vi "Measure.vi"(8 "error in (no error)":errorcluster, 9 "measurement configuration":variant, 10 "measure call context in":refnum<class "Measure Call Context.lvclass">, 11 "measurement plugin in":refnum<class "FPT NoiseFigure.lvclass">) -> (0 "error out":errorcluster, 1 "measurement results":variant, 2 "measure call context out":refnum<class "Measure Call Context.lvclass">, 3 "measurement plugin out":refnum<class "FPT NoiseFigure.lvclass">)   [LabVIEW 2023, in "FPT NoiseFigure.lvclass"]
uses:
  FPT NoiseFigure.lvclass
  <vilib>/Plug-In SDKs/Measurements/Measure Call Context/Measure Call Context.lvclass
  Measurement Configuration.ctl
  FPT NoiseFigure.lvclass/FPT NoiseFigure.ctl
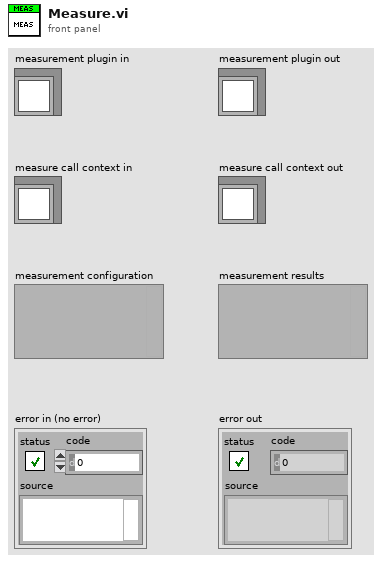
[diagram p1: front panel]
types:
  T1 = typedef "FPT NoiseFigure.lvclass/Measurement Configuration.ctl" = cluster{"Automation Test":bool, "Power sequencing file path":string, "RFmx name":string, "RFmx port":string, "DUT Max Gain (dB)":dbl, "DUT Max Noise Figure (dB)":dbl, "Reference Level Mode":enum32{"Manual", "Recommend"}, "Reference Level (dBm)":dbl, "Preamp Enabled":i32, "RFmx attenuation mode":enum32{"<None>", "Constant Attenuation", "s2p File"}, "RFmx external attenuation (dB)":dbl, "RFmx s-parameters orientation":enum32{"Port1 Towards DUT", "Port2 Towards DUT"}, "RFmx s2p file path":string, "Switch Name":string, "Switch Connection":string, "ENS SMU Name":string, "ENS SMU Channel":string, "Action":u32, "Measurement Bandwidth (Hz)":dbl, "Measurement Interval (s)":dbl, "NF Cal Setup ID":string, "DUT Type":i32, "Frequency List Mode":enum32{"Step", "Points", "Frequency List"}, "Step - Start Frequency ":dbl, "Step - Stop Frequency":dbl, "Step - Step Size":dbl, "Points - Start Frequency":dbl, "Points - Stop Frequency":dbl, "Points - Number of Points":i32, "FreqList - Frequency List":dbl[], "Averaging Enabled":bool, "Averaging Count":i32, "Noise Source Type":i32, "Noise Source RFSG Port":string, "Noise Source Cold Temperature (K)":dbl, "Noise Source Off Temperature (K)":dbl, "ENR Freq (Hz)":dbl[], "ENR (dB)":dbl[], "DUT Input_Compensation Enabled":bool, "DUT Input_Temperation (K)":dbl, "DUT Input_Loss Freq (Hz)":dbl[], "DUT Input_Loss (dB)":dbl[], "DUT Output_Compensation Enabled":bool, "DUT Output_Temperation (K)":dbl, "DUT Output_Loss Freq (Hz)":dbl[], "DUT Output_Loss (dB)":dbl[], "Calibration_Compensation Enabled":bool, "Calibration_Temperation (K)":dbl, "Calibration_Loss Freq (Hz)":dbl[], "Calibration_Loss (dB)":dbl[], "Noise Source_Compensation Enabled":bool, "Noise Source_Temperation (K)":dbl, "Noise Source_Loss Freq (Hz)":dbl[], "Noise Source_Loss (dB)":dbl[], "DUT Input Loss S2P File Path":string, "DUT Input Loss S-Parameter Orientation":i32, "DUT Output Loss S2P File Path":string, "DUT Output Loss S-Parameter Orientation":i32, "Calibration Loss S2P File Path":string, "Calibration Loss S-Parameter Orientation":i32, "Noise Source Loss S2P File Path":string, "Noise Source Loss S-Parameter Orientation":i32, "Power sequencing file validity check":bool}
  T2 = typedef "FPT NoiseFigure.lvclass/Measurement Results.ctl" = cluster{"Status":string, "DUT NF vs Freq":dbl[][], "Analyzer NF vs Freq":dbl[][], "DUT NF (mean)":dbl, "Analyzer NF (mean)":dbl}
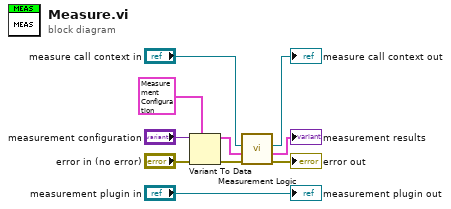
[diagram p0: block diagram]
diagram:
  n1 = Variant To Data(error in="error in (no error)", type=T1 {"Automation Test"=FALSE, "Power sequencing file path"="Lorem ipsum dolor sit", "RFmx name"="5842_0", "RFmx port"="Lorem ipsum dolor sit", "DUT Max Gain (dB)"=3.0, "DUT Max Noise Figure (dB)"=1.2, "Reference Level Mode"=enum."Manual", "Reference Level (dBm)"=1.2, "Preamp Enabled"=0, "RFmx attenuation mode"=enum."Constant Attenuation", "RFmx external attenuation (dB)"=1.0, "RFmx s-parameters orientation"=enum."Port2 Towards DUT", "RFmx s2p file path"="", "Switch Name"="2599_S8", "Switch Connection"="no0->com0", "ENS SMU Name"="", "ENS SMU Channel"="", "Action"=0, "Measurement Bandwidth (Hz)"=4000000.0, "Measurement Interval (s)"=0.1, "NF Cal Setup ID"="SNS_PS_6dB_ENR15_26.5GHz_VI", "DUT Type"=0, "Frequency List Mode"=enum."Step", "Step - Start Frequency "=1000000000.0, "Step - Stop Frequency"=2000000000.0, "Step - Step Size"=100000000.0, "Points - Start Frequency"=1000000000.0, "Points - Stop Frequency"=2000000000.0, "Points - Number of Points"=11, "FreqList - Frequency List"=[4000000000.0, 5000000000.0, 6000000000.0, 7000000000.0, 8000000000.0, 9000000000.0, 10000000000.0, 11000000000.0, 12000000000.0, 13000000000.0, 14000000000.0, 15000000000.0, 16000000000.0, 17000000000.0, 18000000000.0, 19000000000.0, 20000000000.0], "Averaging Enabled"=FALSE, "Averaging Count"=10, "Noise Source Type"=1, "Noise Source RFSG Port"="port1", "Noise Source Cold Temperature (K)"=302.8, "Noise Source Off Temperature (K)"=297.0, "ENR Freq (Hz)"=[6500000000.0], "ENR (dB)"=[15.0], "DUT Input_Compensation Enabled"=FALSE, "DUT Input_Temperation (K)"=297.0, "DUT Input_Loss Freq (Hz)"=array[589 elements], "DUT Input_Loss (dB)"=array[589 elements], "DUT Output_Compensation Enabled"=FALSE, "DUT Output_Temperation (K)"=297.0, "DUT Output_Loss Freq (Hz)"=array[589 elements], "DUT Output_Loss (dB)"=array[589 elements], "Calibration_Compensation Enabled"=FALSE, "Calibration_Temperation (K)"=297.0, "Calibration_Loss Freq (Hz)"=array[589 elements], "Calibration_Loss (dB)"=array[589 elements], "Noise Source_Compensation Enabled"=FALSE, "Noise Source_Temperation (K)"=297.0, "Noise Source_Loss Freq (Hz)"=[], "Noise Source_Loss (dB)"=[], "DUT Input Loss S2P File Path"="", "DUT Input Loss S-Parameter Orientation"=0, "DUT Output Loss S2P File Path"="", "DUT Output Loss S-Parameter Orientation"=0, "Calibration Loss S2P File Path"="", "Calibration Loss S-Parameter Orientation"=0, "Noise Source Loss S2P File Path"="", "Noise Source Loss S-Parameter Orientation"=0, "Power sequencing file validity check"=TRUE} ("measurement configuration"), Variant="measurement configuration") -> (data=w1:T1, error out=w7:errorcluster)
  n2 = call "Measurement Logic.vi"("error in"=w7, "measurement configuration"=w1, "measure call context in"="measure call context in") -> ("error out"=→"error out":errorcluster, "measurement results"=→"measurement results":T2, "measure call context out"=→"measure call context out":refnum<class "Measure Call Context.lvclass">)  [unwired: 6 in]
  "measurement plugin out" <- "measurement plugin in"
